vi "Next Step.vi"(8 "error in (no error)":errorcluster, 11 "Stepper in":refnum<class "Stepper.lvclass">) -> (0 "error out":errorcluster, 3 "Stepper out":refnum<class "Stepper.lvclass">)   [LabVIEW 2021, in "Stepper.lvclass"]
uses:
  Stepper.lvclass
  C:/Git/LabActor/Instrument Actor/Instrument Actor.lvclass
  NHMFL_Core/Libraries/Utilities/Output Value/Output Value.lvclass
  C:/Git/NHMFL_Core/Libraries/Instruments/Results/Acquired Result/Acquired Result.lvclass
  Instrument Actor/Instrument Actor.lvclass/Instrument Actor.ctl
  Instrument Actor/Read Instrument driver.vi
  Instrument Actor/Write Instrument driver.vi
  NHMFL_Core/Libraries/Instruments/Instrument Driver/Instrument Driver.lvclass
  Measurements/Response Synchronizer/Response Synchronizer.lvclass
  Stepper.lvclass/Stepper.ctl
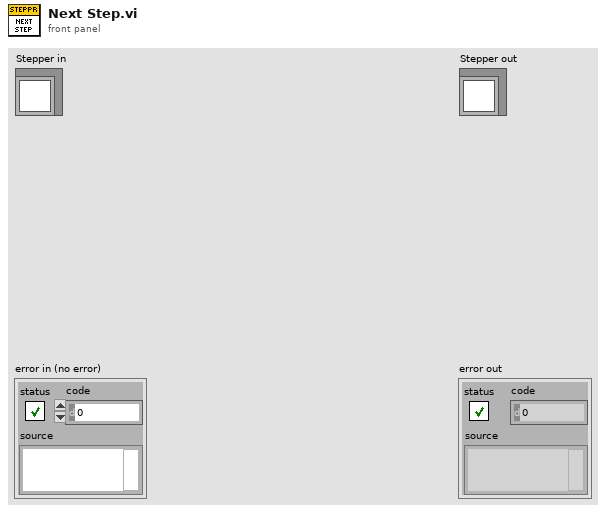
[diagram p1: front panel]
types:
  T1 = typedef "Stepper Config.ctl" = cluster{"Start":dbl, "End":dbl, "Step":dbl, "Append measurements":string[]}
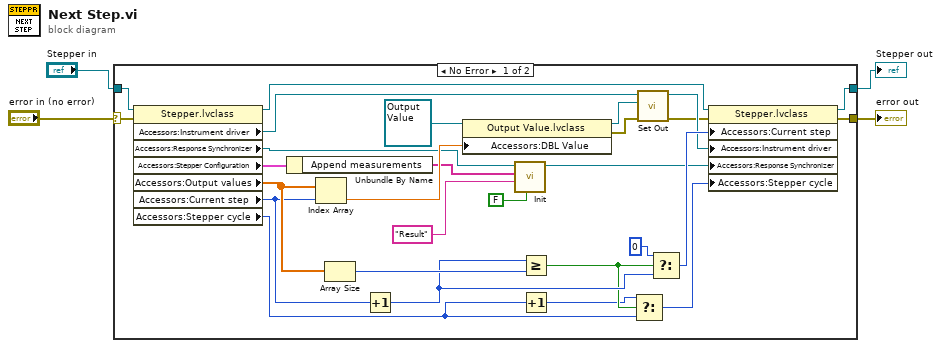
[diagram p0: block diagram]
diagram:
  n1 = case shown="No Error" "error in (no error)" {
    selector: "error in (no error)" -> [w32 w34]
    tunnel: [w9 w34] -> w3
    tunnel: [w24 w33] -> w1
    tunnel: "Stepper in" -> [w31 w33]
    frame No Error {
      n2 = property class="Stepper.lvclass"(reference=w31, error in=w32) -> (reference out=w25:refnum<class "Stepper.lvclass">, "Accessors:Instrument driver"=w23:refnum<class "Instrument Driver.lvclass">, "Accessors:Response Synchronizer"=w15:refnum<class "Response Synchronizer.lvclass">, "Accessors:Stepper Configuration"=w14:T1, "Accessors:Output values"=w27:dbl[], "Accessors:Current step"=w26:i32, "Accessors:Stepper cycle"=w7:i32)  [unwired: 1 out]
      n3 = Unbundle By Name(w14) -> ("Append measurements"=w13:string[])
      n4 = Index Array(array=w27, index=w26) -> (element=w20:dbl)
      n5 = Array Size(array=w27) -> (size(s)=w30:i32)
      n6 = Increment(x=w26) -> (x+1=w29:i32)
      n7 = property class="Output Value.lvclass"(reference=refnum<class "Output Value.lvclass"> refnum ("Output value"), "Accessors:DBL Value"=w20) -> (reference out=w21:refnum<class "Output Value.lvclass">, error out=w16:errorcluster)  [unwired: 1 in]
      n8 = call-dynamic "Init.vi"("Subscribe"=FALSE, "Topic"="Result", "Responder names"=w13, "Response Synchronizer in"=w15) -> ("Response Synchronizer out"=w10:refnum<class "Response Synchronizer.lvclass">)  [unwired: 6 in, 1 out]
      n9 = Greater Or Equal?(x=w29, y=w30) -> (x >= y?=w8:bool)
      n10 = Increment(x=w7) -> (x+1=w6:i32)
      n11 = Select(t=w6, s=w8, f=w7) -> (s? t:f=w5:i32)
      n12 = call-dynamic "Set Out.vi"("error in (no error)"=w16, "Output value"=w21, "Instrument Driver in"=w23) -> ("error out"=w17:errorcluster, "Instrument Driver out"=w18:refnum<class "Instrument Driver.lvclass">)  [unwired: 7 in]
      n13 = Select(t=0, s=w8, f=w29) -> (s? t:f=w19:i32)
      n14 = property class="Stepper.lvclass"(reference=w25, error in=w17, "Accessors:Current step"=w19, "Accessors:Instrument driver"=w18, "Accessors:Response Synchronizer"=w10, "Accessors:Stepper cycle"=w5) -> (reference out=w24:refnum<class "Stepper.lvclass">, error out=w9:errorcluster)
    }
    frame Error {
    }
  }
  "error out" <- w3
  "Stepper out" <- w1
